vi "Data.vi"(11 "Data Queue":refnum<queue>) -> ()   [LabVIEW 2013, in "main.lvlib"]
uses:
  main.lvlib
  Controls/Reference AE Control.ctl
  Controls/Enum Variables.ctl
  Data Processing/ProcessData(SubVI).vi
panel:
  in  "StopBtn":bool=TRUE
  out "cmString":string="cm" caption="CMString"
  out "AdjustedHeight":dbl caption="Højdejustering"
  in  "FilterControl":bool caption="Filter"
  in  "Tangent On/Off":bool caption="Deactivate Tangents"
  in  "ProcessDataTreeMenu":string(tree)
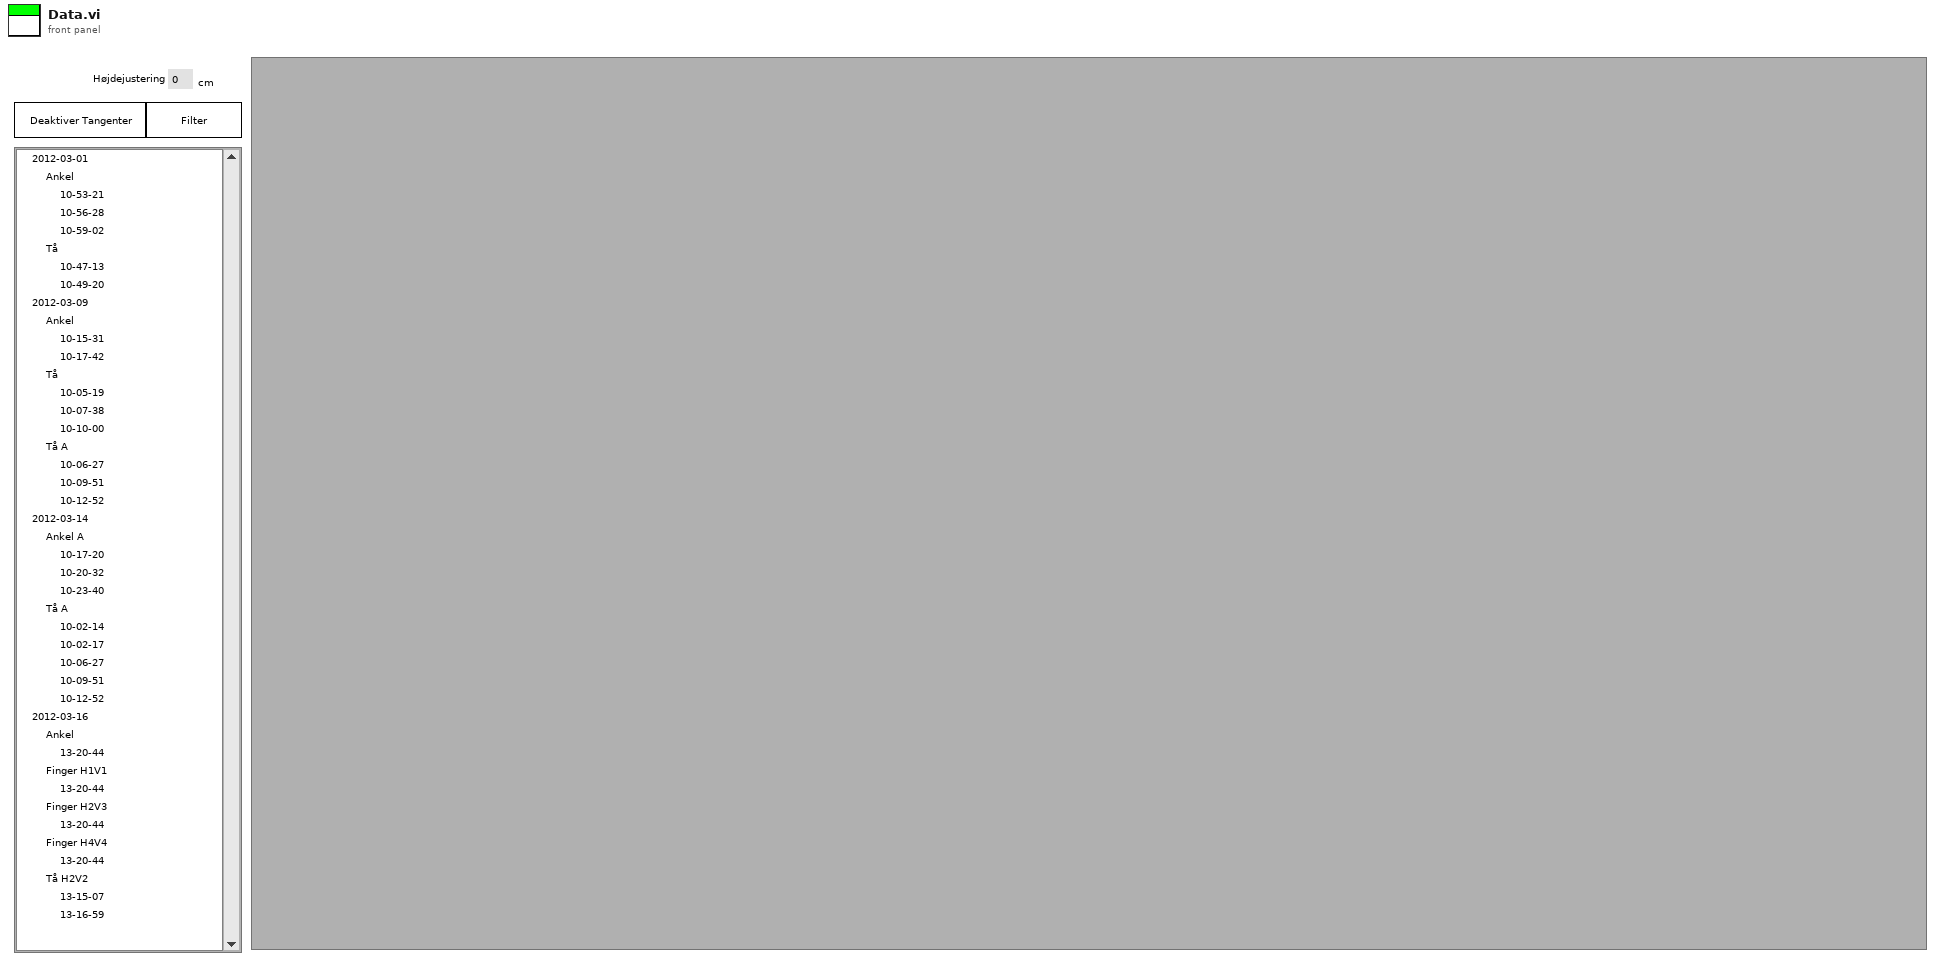
[diagram p1: front panel]
types:
  T1 = typedef "main.lvlib/Reference AE Control.ctl" = enum16{"Initialize", "Set Menu", "Set Profile", "Set Configuration", "Set Configuration_old", "Set Configuration_new", "Set Configuration Method", "Set Acquisition", "Set Data", "Set Journal", "Get"}
  T2 = typedef "main.lvlib/Enum Variables.ctl" = enum16{"SetAcqFilter", "GetAcqFilter", "Set Filter", "Get Filter", "Set Height", "Get Height", "Set Recorded Height", "Get Recorded Height", "Set Blue Pressure", "Get Blue Pressure", "Set Red Pressure", "Get Red Pressure", "Init", "Reset Pressure", "Set Red Cursors", "Get Red Cursors", "Set Blue Cursors", "Get Blue Cursors", "Set Language", "Get Language", "Set Active Graphs", "Get ActiveGraphs", "Set Method", "Get Method", "Set Encryption", "Get Encryption", "Set ExcelVersion", "Get ExcelVersion", "Set DICOM Avail", "Get DICOM Avail", "Set DICOM Encode", "Get DICOM Encode", "Set JournalExport", "Get JournalExport", "Set Sequence", "Get Sequence", "Set DAQ Connected", "Get DAQ Connected", "Set Current Graph", "Get Current Graph", "Set General Settings", "Get Hyphenation", "Set Arm Calc Method", "Get Arm Calc Method", "Set Dicom Tags", "Get Dicom Tags", "Set BT Serial", "Get BT Serial", "Set BT Accepted Serials", "Get BT Accepted Serials", "Get BT License", "Set BT License"}
  T3 = cluster{"cmString":refnum<vi>, "AdjustedHeight":refnum<vi>, "ProcessDataTreeMenu":refnum<vi>, "Tangent On/Off":refnum<vi>, "FilterControl":refnum<vi>}
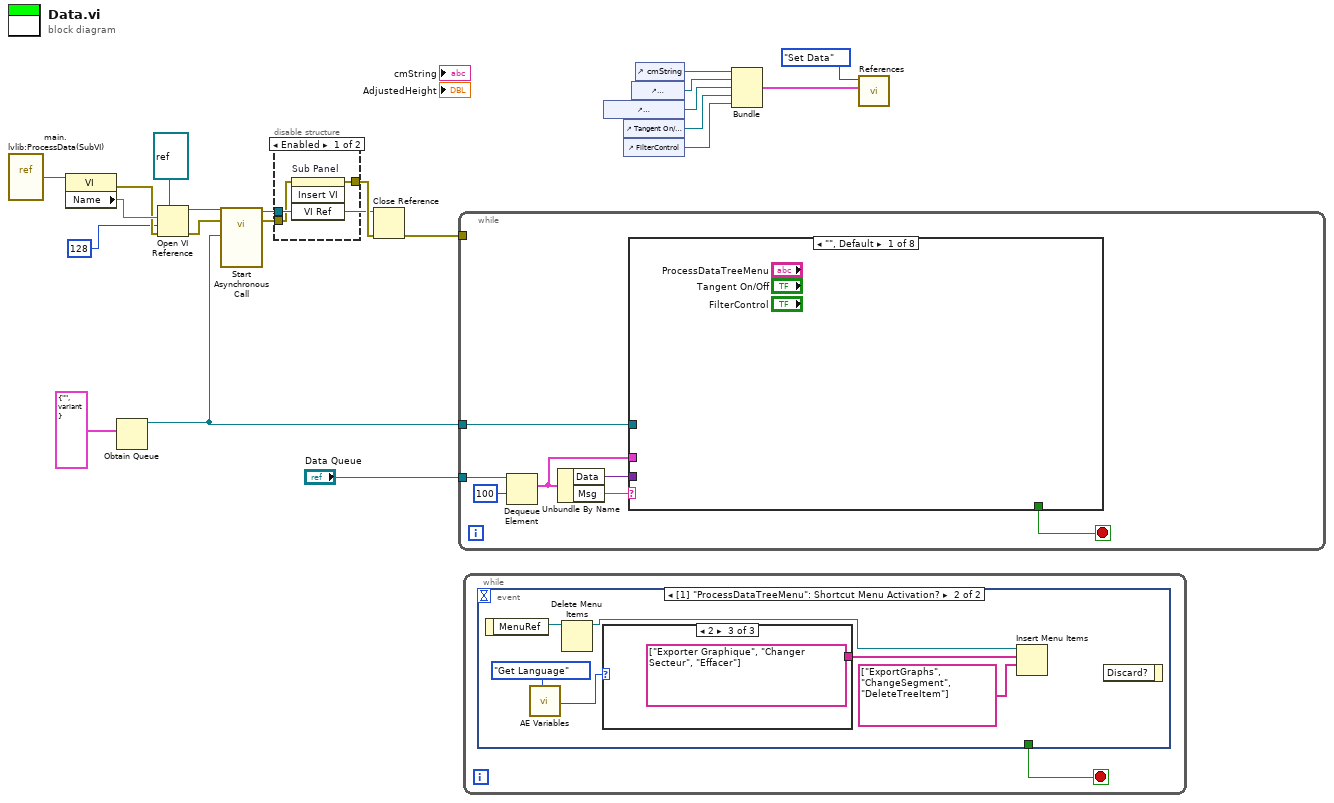
[diagram p0: block diagram]
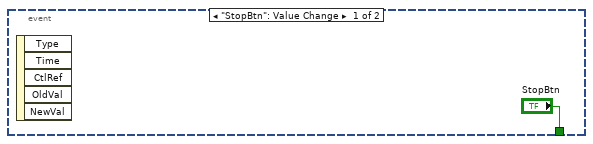
[diagram p3: hidden frame]
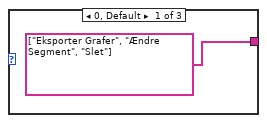
[diagram p4: hidden frame]
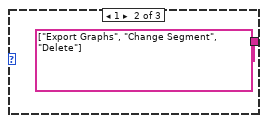
[diagram p5: hidden frame]
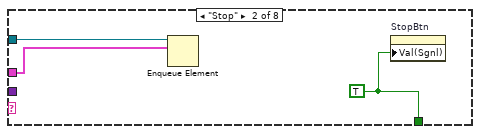
[diagram p6: hidden frame]
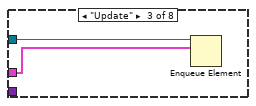
[diagram p7: hidden frame]
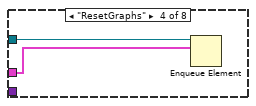
[diagram p8: hidden frame]
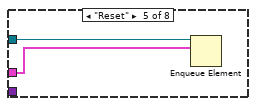
[diagram p9: hidden frame]
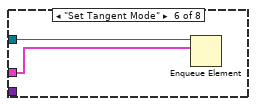
[diagram p10: hidden frame]
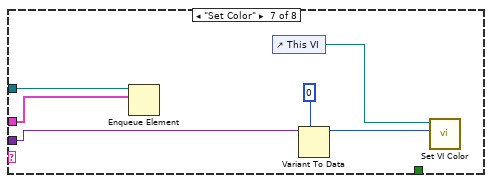
[diagram p11: hidden frame]
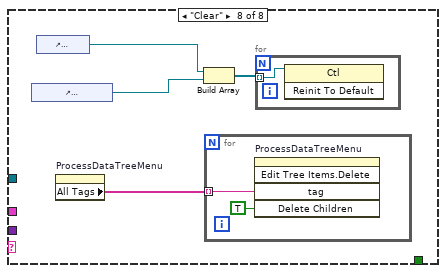
[diagram p12: hidden frame]
diagram:
  n1 = vi-ref "main.lvlib:ProcessData(SubVI).vi"() -> (w13:refnum<vi>)
  n2 = property class="VI"(reference=w13) -> (error out=w6:errorcluster, "Name"=w12:string)  [unwired: 1 in, 1 out]
  n3 = Obtain Queue(element data type=cluster{"Msg":string, "Data":variant} {"Msg"="", "Data"=variant}) -> (queue out=w3:refnum<queue>)  [unwired: 4 in, 2 out]
  n4 = Open VI Reference(type specifier VI Refnum (for type only)=refnum<vi> refnum ("application reference (local)"), vi path=w12, options=128, error in (no error)=w6) -> (vi reference=w10:refnum<vi>, error out=w7:errorcluster)  [unwired: 2 in]
  n5 = call-by-ref "Start Asynchronous Call"(reference=w10, error in=w7, "Queue"=w3) -> (reference out=w5:refnum<vi>, error out=w8:errorcluster)  [unwired: 5 in]
  n6 = disable-structure shown="Enabled" {
    disable-tunnel: [w24 w25] -> w9
    disable-tunnel: w8 -> [w23 w25]
    disable-tunnel: w5 -> [w22 _]
    frame Enabled {
      n7 = invoke on="Sub Panel" class="SubPanel" method="Insert VI"(error in=w23, "VI Ref"=w22) -> (error out=w24:errorcluster)  [unwired: 2 in, 3 out]
    }
    frame Disabled {
    }
  }
  n8 = Close Reference(reference=w5, error in (no error)=w9) -> (error out=w4:errorcluster)
  n9 = while {
    tunnel: "Data Queue" -> [w32]
    tunnel: w4 -> [_]
    tunnel: w3 -> [w29]
    stop <- w30 stop-if-true
    n10 = Dequeue Element(queue=w32, timeout in ms (-1)=100) -> (element=w26:cluster{"Msg":string, "Data":variant})  [unwired: 1 in, 3 out]
    n11 = Unbundle By Name(w26) -> ("Data"=w27:variant, "Msg"=w31:string)
    n12 = case shown="\"\", Default" w31 {
      tunnel: [_ w33 _ _ _ _ _ _] -> w30
      tunnel: w29 -> [_ w35 w37 w39 w41 w43 w45 _]
      tunnel: w27 -> [_ _ _ _ _ _ w46 _]
      tunnel: w26 -> [_ w34 w36 w38 w40 w42 w44 _]
      frame "", Default {
      }
      frame "Stop" {
        w33 = TRUE
        n13 = Enqueue Element(queue=w35, element=w34) -> ()  [unwired: 2 in, 3 out]
        n14 = property on="StopBtn" class="Bool (strict)"("Val(Sgnl)"=w33) -> ()  [unwired: 2 in, 2 out]
      }
      frame "Update" {
        n15 = Enqueue Element(queue=w37, element=w36) -> ()  [unwired: 2 in, 3 out]
      }
      frame "ResetGraphs" {
        n16 = Enqueue Element(queue=w39, element=w38) -> ()  [unwired: 2 in, 3 out]
      }
      frame "Reset" {
        n17 = Enqueue Element(queue=w41, element=w40) -> ()  [unwired: 2 in, 3 out]
      }
      frame "Set Tangent Mode" {
        n18 = Enqueue Element(queue=w43, element=w42) -> ()  [unwired: 2 in, 3 out]
      }
      frame "Set Color" {
        n19 = Enqueue Element(queue=w45, element=w44) -> ()  [unwired: 2 in, 3 out]
        n20 = control-ref of="This VI"() -> (w49:refnum<vi>)
        n21 = Variant To Data(type=u32 0 ("Pane Color"), Variant=w46) -> (data=w47:u32)  [unwired: 1 in, 1 out]
        n22 = call "Set VI Color.vi"("Pane Color"=w47, "VI in"=w49) -> ()  [unwired: 10 in]
      }
      frame "Clear" {
        n23 = control-ref of="ProcessDataTreeMenu"() -> (w51:refnum<vi>)
        n24 = control-ref of="AdjustedHeight"() -> (w52:refnum<vi>)
        n25 = property on="ProcessDataTreeMenu" class="Tree (strict)"() -> ("All Tags"=w53:string[])  [unwired: 2 in, 2 out]
        n26 = Build Array(w52, w51) -> (w50:refnum<vi>[])
        n27 = for {
          tunnel: w53 -> [w55] mode=indexing
          n28 = invoke on="ProcessDataTreeMenu" class="Tree (strict)" method="Edit Tree Items.Delete"("tag"=w55, "Delete Children"=TRUE ("Delete Children?")) -> ()  [unwired: 3 in, 5 out]
        }
        n29 = for {
          tunnel: w50 -> [w56] mode=indexing
          n30 = invoke class="Ctl" method="Reinit To Default"(reference=w56) -> ()  [unwired: 2 in, 3 out]
        }
      }
    }
  }
  n31 = while {
    stop <- w57 stop-if-true
    n32 = event shown="[1] \"ProcessDataTreeMenu\": Shortcut Menu Activation?" {
      selector: _ -> [_ _]
      dyn-events: _ -> [_ _]
      timeout: _ -> [_ _]
      tunnel: ["StopBtn" _] -> w57
      event "StopBtn": Value Change {
        n33 = event-data() -> ()  [unwired: 1 in, 5 out]
      }
      event "ProcessDataTreeMenu": Shortcut Menu Activation? {
        n34 = event-data() -> ("MenuRef"=w64:refnum<k9>)  [unwired: 1 in]
        n35 = call "AE Variables.vi"("Action"=Enum_Variables."Get Language") -> ("RingOut"=w59:u16)  [unwired: 11 in, 7 out]
        n36 = Delete Menu Items(9:w64) -> (3:w61:refnum<k9>)  [unwired: 3 in, 1 out]
        n37 = case shown="2" w59 {
          tunnel: [string[] ["Eksporter Grafer", "Ændre Segment", "Slet"] string[] ["Export Graphs", "Change Segment", "Delete"] string[] ["Exporter Graphique", "Changer Secteur", "Effacer"]] -> w62
          frame 0, Default {
          }
          frame 1 {
          }
          frame 2 {
          }
        }
        n38 = Insert Menu Items(7:string[] ["ExportGraphs", "ChangeSegment", "DeleteTreeItem"] ("item tags"), 8:w62, 9:w61) -> ()  [unwired: 3 in, 3 out]
        n39 = event-data() -> ()  [unwired: 2 in, 1 out]
      }
    }
  }
  n40 = control-ref of="ProcessDataTreeMenu"() -> (w19:refnum<vi>)
  n41 = control-ref of="Tangent On/Off"() -> (w18:refnum<vi>)
  n42 = control-ref of="FilterControl"() -> (w17:refnum<vi>)
  n43 = control-ref of="AdjustedHeight"() -> (w20:refnum<vi>)
  n44 = control-ref of="cmString"() -> (w21:refnum<vi>)
  n45 = Bundle("cmString"=w21, "AdjustedHeight"=w20, "ProcessDataTreeMenu"=w19, "Tangent On/Off"=w18, "FilterControl"=w17) -> (w16:T3)  [unwired: 1 in]
  n46 = call "References.vi"("variant"=w16, "Reference AE Control"=Reference_AE_Control."Set Data") -> ()  [unwired: 8 in, 2 out]
